vi "S7.vi"   [LabVIEW 2020]
uses:
  S7Ref.vi
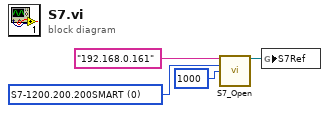
[diagram p0: block diagram]
diagram:
  w3 = u8 0 items=["S7-1200.200.200SMART"=0, "S7-300"=2, "S7-400"=3] ("PLC 系列")
  n1 = call "S7_Open.vi"("IP 地址"="192.168.0.161", "PLC 系列"=w3, "超时（MS）"=1000) -> ("TCP"=w1:refnum<k5>)  [unwired: 10 in, 2 out]
  n2 = global write "S7Ref.vi" "S7Ref"(w1) -> ()
